vi "set_config_cluster.vi"(8 "error in (no error)":errorcluster, 10 "config cluster variant":variant, 11 "SegmenterDL100224ThreeD in":refnum<class "SegmenterDL100224ThreeD.lvclass">) -> (0 "error out":errorcluster, 3 "SegmenterDL100224ThreeD out":refnum<class "SegmenterDL100224ThreeD.lvclass">)   [LabVIEW 2010, in "SegmenterDL100224ThreeD.lvclass"]
uses:
  SegmenterDL100224ThreeD.lvclass
  SegmenterDL100224ThreeD.lvclass/SegmenterDL100224ThreeD.ctl
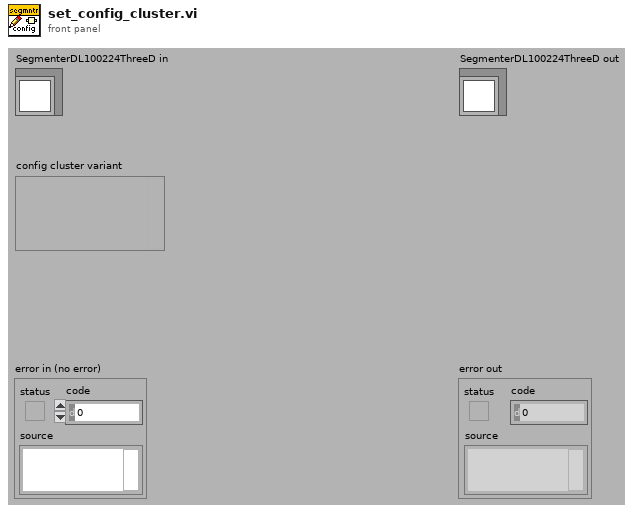
[diagram p1: front panel]
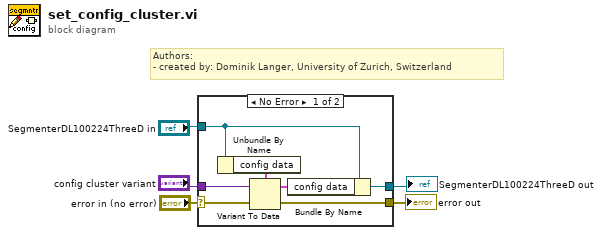
[diagram p0: block diagram]
diagram:
  # "Authors: \n- created by: Dominik Langer, University of Zurich, Switzerland"
  n1 = case shown="No Error" "error in (no error)" {
    selector: "error in (no error)" -> [w10 w13]
    tunnel: "SegmenterDL100224ThreeD in" -> [w8 w14]
    tunnel: [w7 w13] -> w1
    tunnel: [w6 w14] -> w2
    tunnel: "config cluster variant" -> [w9 _]
    frame No Error {
      n2 = Unbundle By Name(w8) -> ("config data"=w12:cluster{"preprocessing macro":string})
      n3 = Variant To Data(error in=w10, Variant=w9, type=w12) -> (error out=w7:errorcluster, data=w11:cluster{"preprocessing macro":string})
      n4 = Bundle By Name(cluster=w8, "config data"=w11) -> (w6:refnum<class "SegmenterDL100224ThreeD.lvclass">)
    }
    frame Error {
    }
  }
  "error out" <- w1
  "SegmenterDL100224ThreeD out" <- w2
